vi "DecodeEnemyState.vi"(8 "error in (no error)":errorcluster, 9 "array":u8[](array[numeric])) -> (0 "error out":errorcluster, 1 "array w/ subset deleted out":u8[](array[numeric]), 3 "output cluster":T2)   [LabVIEW 2017]
uses:
  Core/AI Ball.ctl
panel:
  out "array 2":u8[](array[numeric])
  in  "Cluster":T2
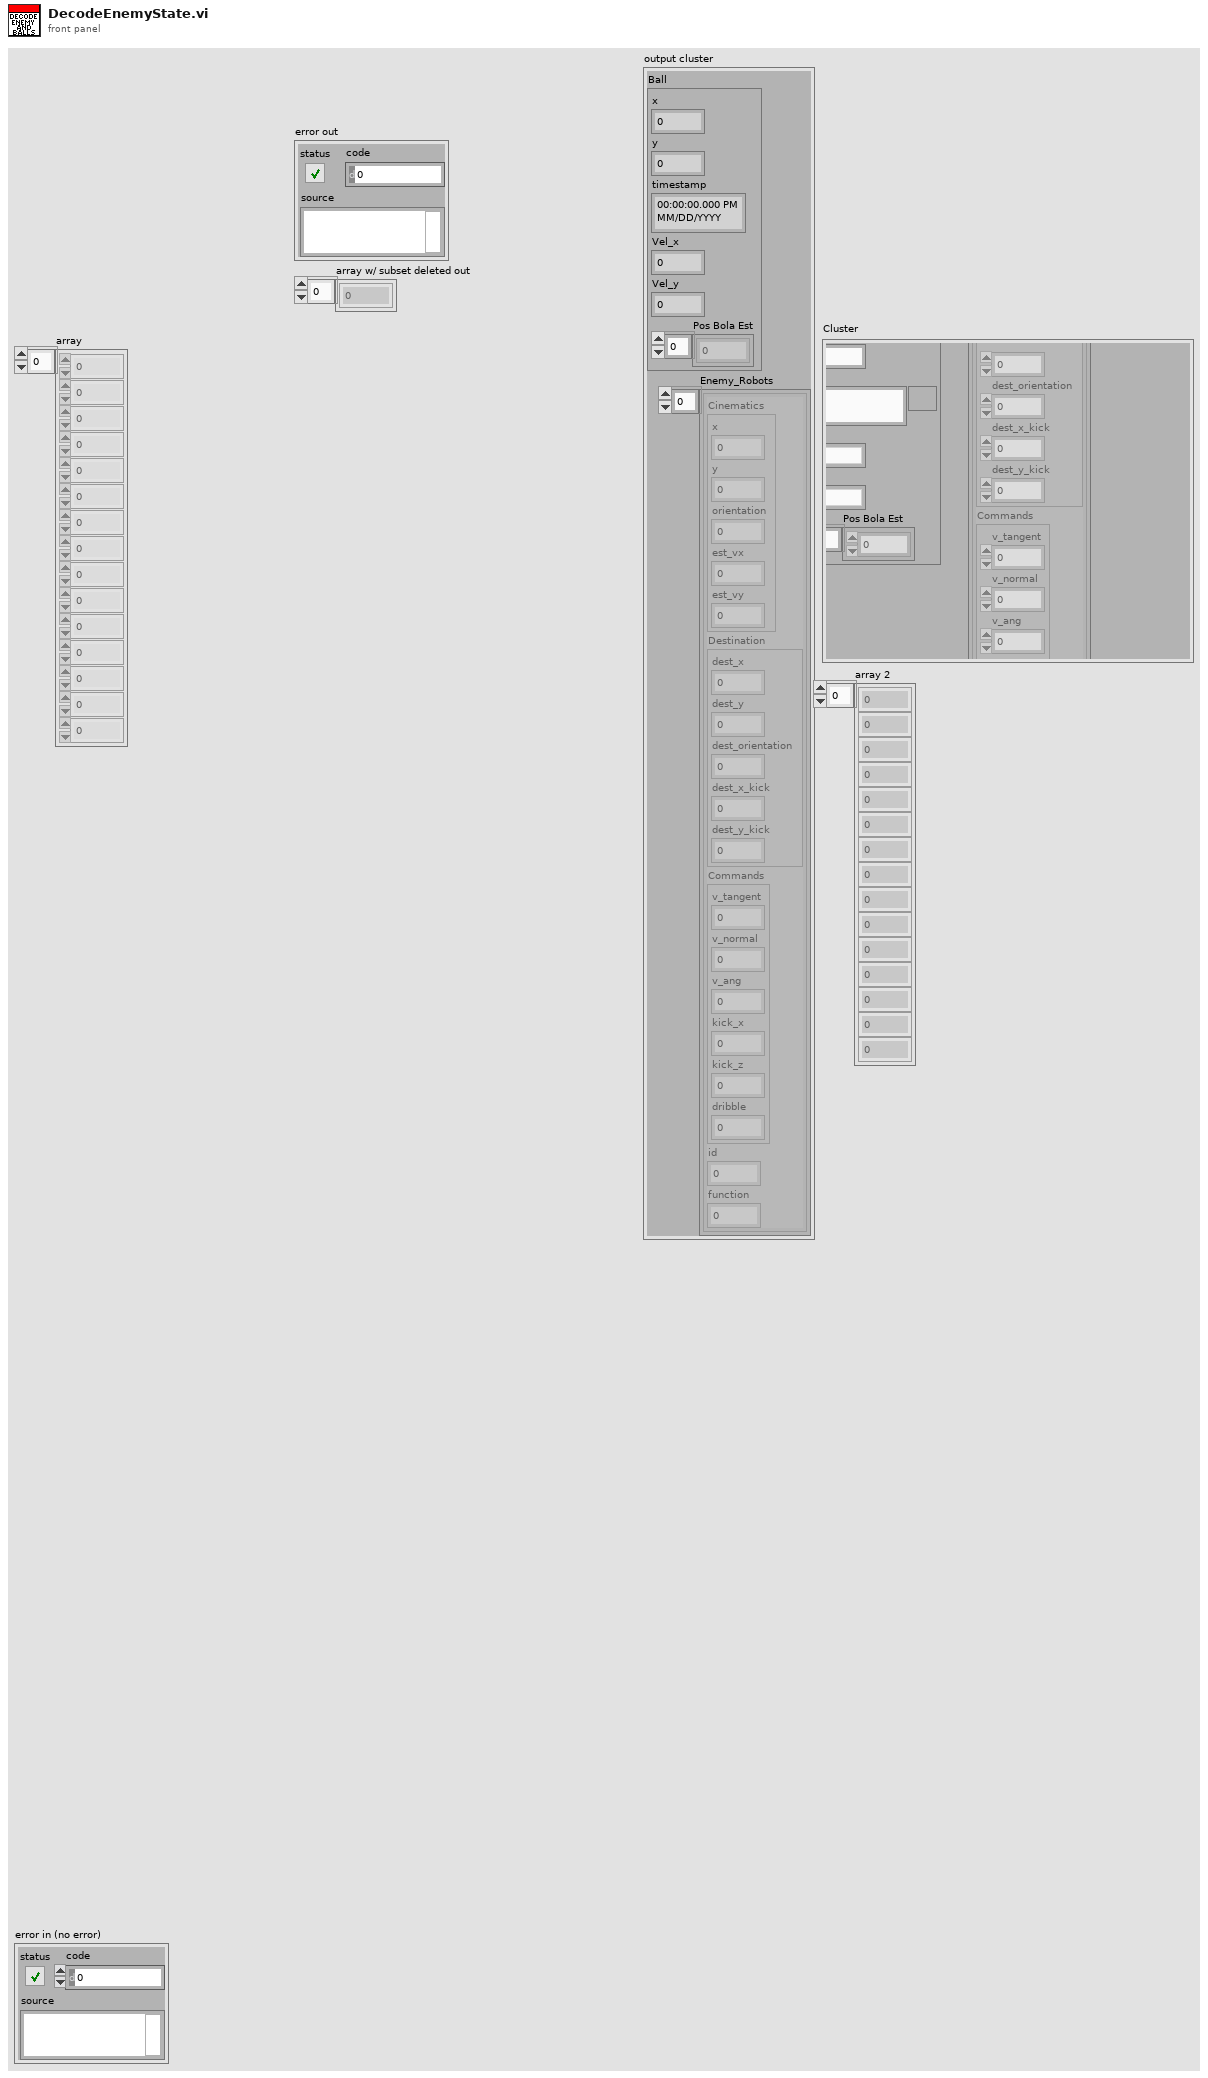
[diagram p1: front panel]
types:
  T1 = typedef "AI Ball.ctl" = cluster{"x":dbl, "y":dbl, "timestamp":timestamp, "Vel_x":dbl, "Vel_y":dbl, "Pos Bola Est":dbl[]}
  T2 = cluster{"Ball":T1, "Enemy_Robots":cluster{"Cinematics":cluster{"x":dbl, "y":dbl, "orientation":dbl, "est_vx":dbl, "est_vy":dbl}, "Destination":cluster{"dest_x":dbl, "dest_y":dbl, "dest_orientation":dbl, "dest_x_kick":dbl, "dest_y_kick":dbl}, "Commands":cluster{"v_tangent":dbl, "v_normal":dbl, "v_ang":dbl, "kick_x":dbl, "kick_z":dbl, "dribble":u32}, "id":u32, "function":u32}[]}
  T3 = cluster{"Cinematics":cluster{"x":dbl, "y":dbl, "orientation":dbl, "est_vx":dbl, "est_vy":dbl}, "Destination":cluster{"dest_x":dbl, "dest_y":dbl, "dest_orientation":dbl, "dest_x_kick":dbl, "dest_y_kick":dbl}, "Commands":cluster{"v_tangent":dbl, "v_normal":dbl, "v_ang":dbl, "kick_x":dbl, "kick_z":dbl, "dribble":u32}, "id":u32, "function":u32}[]
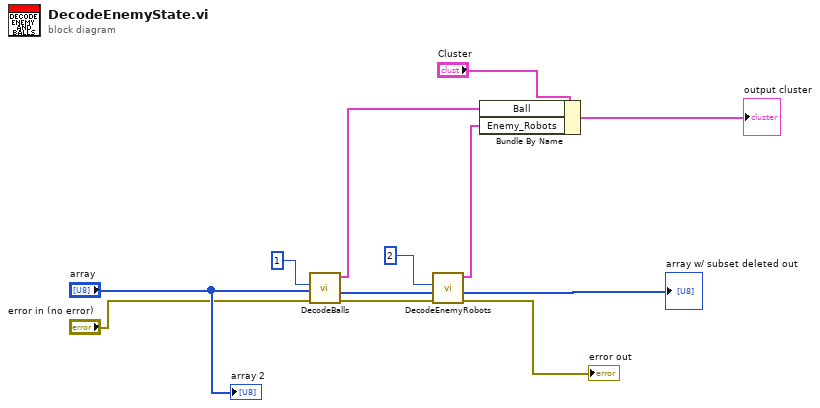
[diagram p0: block diagram]
diagram:
  n1 = call "DecodeBalls.vi"("error in"="error in (no error)", "array"="array", "Key"=1) -> ("error out"=w6:errorcluster, "array w/ subset deleted out"=w7:u8[], "ball"=w3:T1)  [unwired: 6 in]
  n2 = call "DecodeEnemyRobots.vi"("error in"=w6, "array"=w7, "Key"=2) -> ("error out"=→"error out":errorcluster, "array w/ subset deleted out"=→"array w/ subset deleted out":u8[], "Enemy_Robots"=w2:T3)  [unwired: 6 in]
  n3 = Bundle By Name(cluster="Cluster", "Ball"=w3, "Enemy_Robots"=w2) -> (→"output cluster":T2)
  "array 2" <- "array"
